vi "Find All.vi"() -> ()   [LabVIEW 2015]
uses:
  <vilib>/Instr/_visa.llb/VISA Find Search Mode.ctl
  <instrlib>/Fluke 2625A/Fluke 2625A.lvlib
panel:
  out "find list":string[](array[string])
  in  "error in (no error)":errorcluster
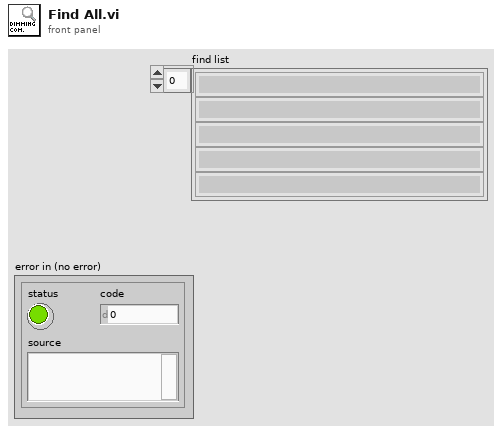
[diagram p1: front panel]
types:
  T1 = typedef "VISA Find Search Mode.ctl" = u32
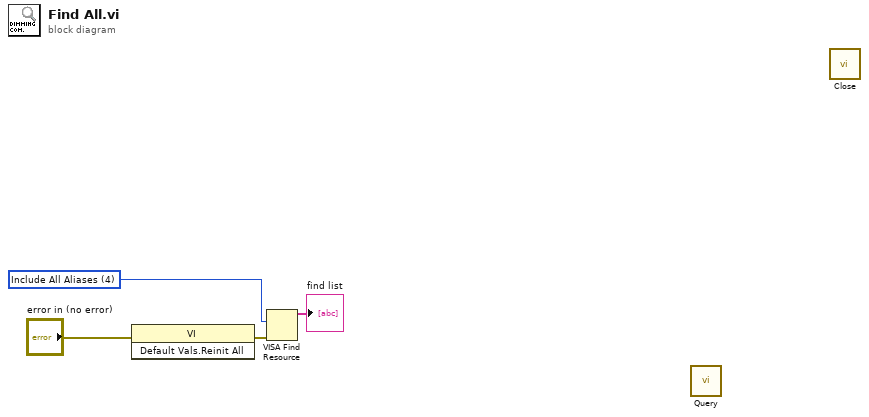
[diagram p0: block diagram]
diagram:
  w4 = T1 4 items=["Canonical Names Only"=0, "Aliases Only"=2, "Include Matching Aliases"=3, "Include All Aliases"=4] ("Search Mode")
  n1 = invoke class="VI" method="Default Vals.Reinit All"(error in="error in (no error)") -> (error out=w2:errorcluster)  [unwired: 2 in, 2 out]
  n2 = VISA Find Resource(8:w2, 10:w4) -> (3:→"find list":string[])  [unwired: 1 in, 2 out]
  n3 = call "Query.vi"() -> ()  [unwired: 18 in, 2 out]
  n4 = call <instrlib>:"Close.vi"() -> ()  [unwired: 11 in, 1 out]
